vi "Read MXN.vi"(8 "error in (no error)":errorcluster, 11 "Bakery Actor in":refnum<class "Bakery Actor.lvclass">) -> (0 "error out":errorcluster, 2 "MXN":bool, 3 "Bakery Actor out":refnum<class "Bakery Actor.lvclass">)   [LabVIEW 2019, in "Bakery Actor.lvlib" / "Bakery Actor.lvclass"]
uses:
  Bakery Actor.lvclass
  Bakery Actor.lvclass/Bakery Actor.ctl
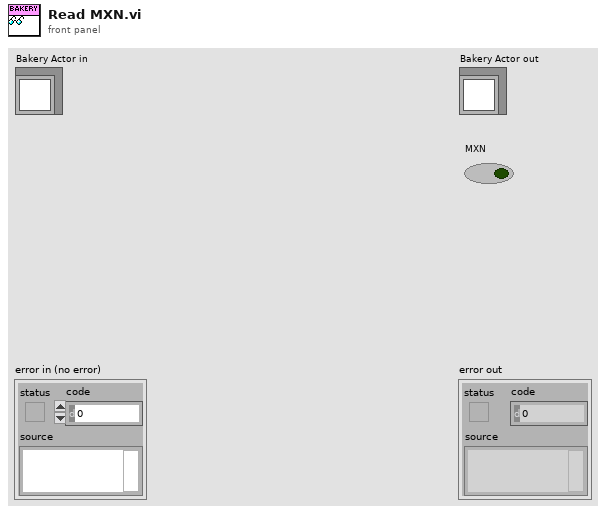
[diagram p1: front panel]
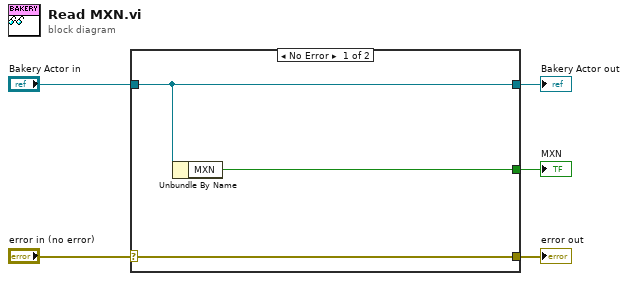
[diagram p0: block diagram]
diagram:
  n1 = case shown="No Error" "error in (no error)" {
    selector: "error in (no error)" -> [w8 w9]
    tunnel: [w8 w9] -> w4
    tunnel: [w7 w10] -> w2
    tunnel: "Bakery Actor in" -> [w7 w10]
    tunnel: [w6 _] -> w1
    frame No Error {
      n2 = Unbundle By Name(w7) -> ("MXN"=w6:bool)
    }
    frame Error {
    }
  }
  "error out" <- w4
  "Bakery Actor out" <- w2
  "MXN" <- w1
